vi "Error handler.vi"(8 "error in":errorcluster) -> (0 "error out":errorcluster, 2 "status":bool, 3 "Status string":string)   [LabVIEW 2014]
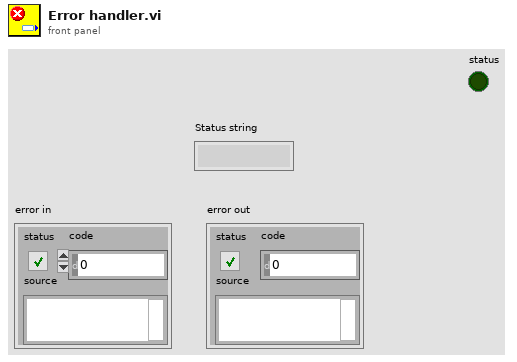
[diagram p1: front panel]
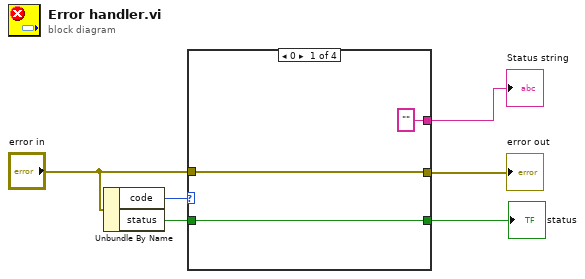
[diagram p0: block diagram]
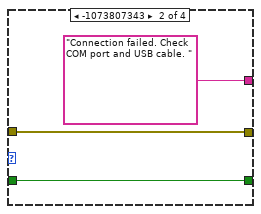
[diagram p2: hidden frame]
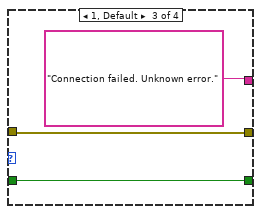
[diagram p3: hidden frame]
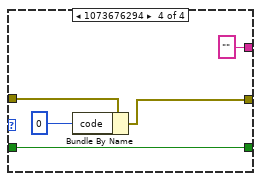
[diagram p4: hidden frame]
diagram:
  n1 = Unbundle By Name("error in") -> ("code"=w6:i32, "status"=w2:bool)
  n2 = case shown="0" w6 {
    tunnel: "error in" -> [w9 w12 w15 w20]
    tunnel: [w9 w12 w15 w19] -> w5
    tunnel: ["" "Connection failed. Check COM port and USB cable. " "Connection failed. Unknown error." ""] -> w3
    tunnel: [w7 w10 w13 w16] -> w1
    tunnel: w2 -> [w7 w10 w13 w16]
    frame 0 {
    }
    frame -1073807343 {
    }
    frame 1, Default {
    }
    frame 1073676294 {
      n3 = Bundle By Name(cluster=w20, "code"=0) -> (w19:errorcluster)
    }
  }
  "error out" <- w5
  "Status string" <- w3
  "status" <- w1
